vi "SaveDataFile.vi"(0 "Data Array":dbl[][](array[numeric])=[[1.0, 1.5e-10, 0.0, 0.0, 0.0], [2.0, 1.5e-10, 0.0, 0.0, 0.0], [3.0, 1.5e-10, 0.0, 0.0, 0.0], [4.0, 1.5e-10, 0.0, 0.0, 0.0]], 1 "Temperature":dbl=18.162352941176472, 3 "Humidity":dbl=25.207500000000007, 5 "no. of arrays":i32=5, 9 "Actual array lengths":i32=4, 11 "Error In":errorcluster, 12 "Array Titles":string="ProbeplanIndex Current PinholeFlag Capacitance Resistance", 13 "Strip Segment":string="Segment\t3T", 14 "Arrays format":string="%^g") -> (4 "Filename OUT":string="c-b1_Striptest_Segment_3T_1.dat", 6 "Pathname OUT":string="c:\\Users\\itk\\Documents\\itk-strip-sensor-data\\R0\\d\\c\\c-b1\\Striptest\\", 10 "Path + Filename OUT":string="c:\\Users\\itk\\Documents\\itk-strip-sensor-data\\R0\\d\\c\\c-b1\\Striptest\\c-b1_Striptest_Segment_3T_1.dat", 15 "Error Out":errorcluster)   [LabVIEW 2018]
uses:
  globals/QC_RunInformation.vi
  <vilib>/regexp/Match Regular Expression.xnode
panel:
  out "Data Array 3":dbl[](array[numeric])
  out "Data Array 2":dbl[](array[numeric])
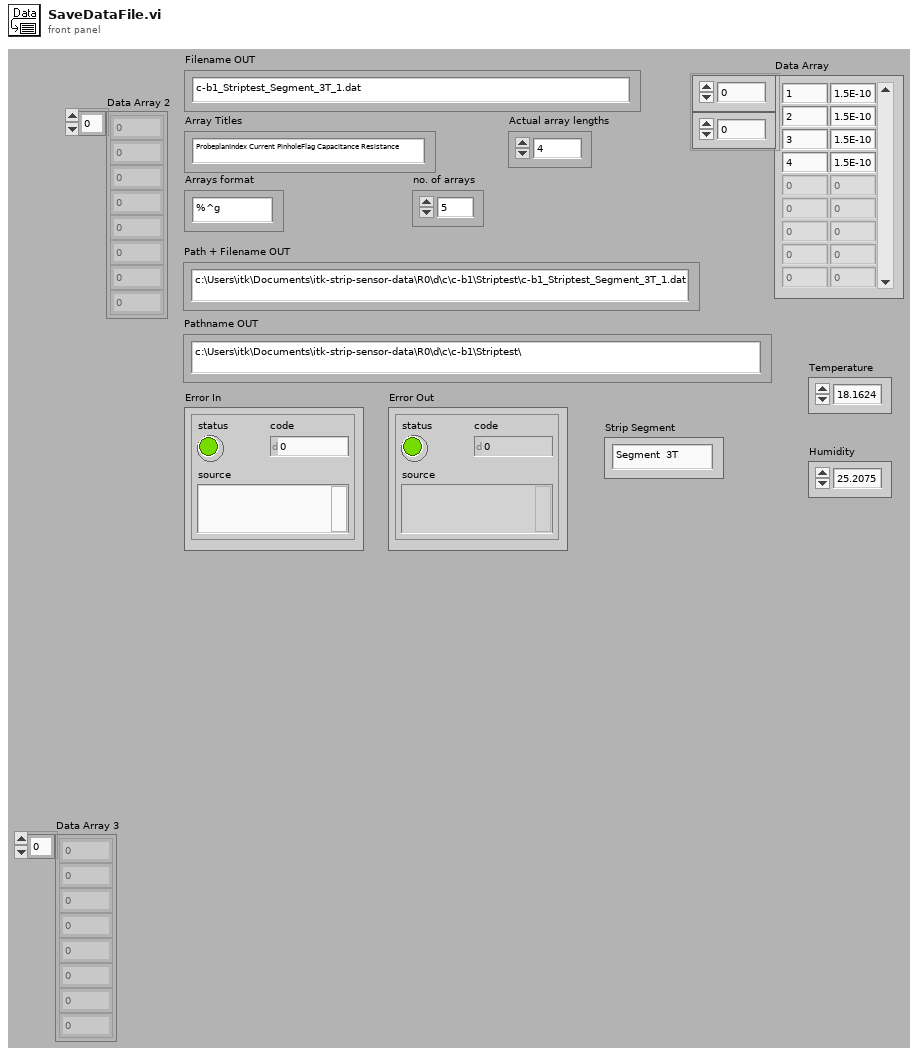
[diagram p1: front panel]
types:
  T1 = enum16{"open", "open or create", "create or replace", "create"}
  T2 = cluster{"Sensor Serial No.:":string, "Wafer Serial No.:":string, "Batch:":string, "Manufacturer:":string, "Device Category:":string, "Database Serial No.:":string, "Initiated:":string, "Test":string, "Instruments used:":string, "Probeplan used:":string, "End of Run comment:":string, "User:":string}
  T3 = cluster{"Institute":string, "Manufacturers":string[], "Devices":string[], "Serialnumbers Lookup DB":string, "Data directory":string, "Backup & screenshot directory":string, "List of known users":string[]}
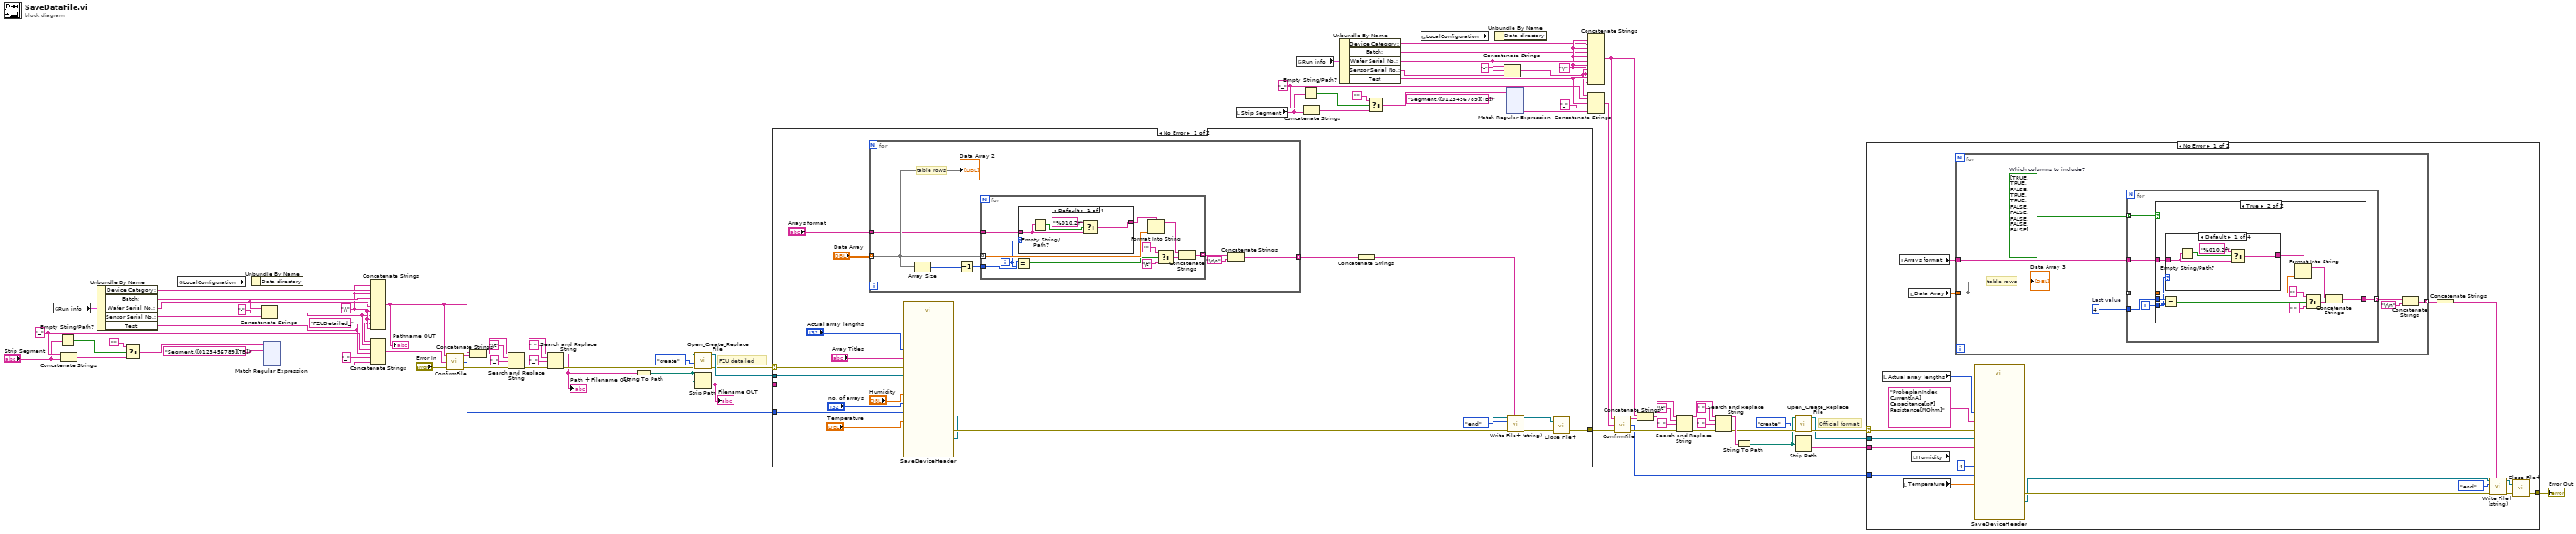
[diagram p0: block diagram]
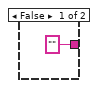
[diagram p2: hidden frame]
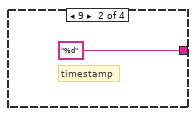
[diagram p3: hidden frame]
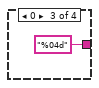
[diagram p4: hidden frame]
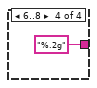
[diagram p5: hidden frame]
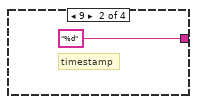
[diagram p7: hidden frame]
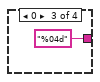
[diagram p8: hidden frame]
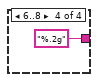
[diagram p9: hidden frame]
diagram:
  w29 = "_"
  w19 = "\\"
  w63 = "_"
  w72 = "\\"
  # "FZU detailed"
  # "Official format"
  n1 = global read "QC_RunInformation.vi" "Run info"() -> (w81:T2)
  n2 = Empty String/Path?(string/path="Strip Segment") -> (empty?=w65:bool)
  n3 = Concatenate Strings(w63, "Strip Segment") -> (w61:string)
  n4 = Unbundle By Name(w81) -> ("Device Category:"=w79:string, "Batch:"=w78:string, "Wafer Serial No.:"=w70:string, "Sensor Serial No.:"=w69:string, "Test"=w4:string)
  n5 = Select(t="", s=w65, f=w61) -> (s? t:f=w48:string)
  n6 = global read "QC_RunInformation.vi" "LocalConfiguration"() -> (w82:T3)
  n7 = Unbundle By Name(w82) -> ("Data directory"=w80:string)
  n8 = Concatenate Strings(w70, "-", w69) -> (w68:string)
  n9 = xnode "Match Regular Expression"("input string"=w48, "regular expression"="Segment.([0123456789][TB])") -> ("submatch 1"=w47:string)  [unwired: 4 in, 5 out]
  n10 = Concatenate Strings(w80, w72, w79, w72, w78, w72, w70, w72, w68, w72, w4, w72) -> (w66:string)
  "Pathname OUT" <- w66
  n11 = Concatenate Strings("FZUDetailed_" ("string"), w68, w63, w4, "_" ("string"), w47) -> (w67:string)
  n12 = call "ConfirmFile.vi"("Error In"="Error In", "Filename IN"=w67, "Pathname IN"=w66) -> ("Error Out"=w56:errorcluster, "RunNr"=w45:i32, "Filename:"=w60:string)
  n13 = Concatenate Strings(w66, w60) -> (w59:string)
  n14 = Search and Replace String(input string=w59, search string="\t" ("string"), replace string="_" ("substring (\"\")"), error in=w56) -> (result string=w53:string, error out=w55:errorcluster)  [unwired: 4 in, 2 out]
  n15 = Search and Replace String(input string=w53, search string=" " ("substring (\"\")"), replace string="_" ("substring (\"\")"), error in=w55) -> (result string=w52:string, error out=w54:errorcluster)  [unwired: 4 in, 2 out]
  "Path + Filename OUT" <- w52
  n16 = String To Path(string=w52) -> (path=w74:path)
  n17 = call <vilib>:"Open_Create_Replace File.vi"("error in (no error)"=w54, "function (open:0)"=T1."create", "file path"=w74) -> ("error out"=w73:errorcluster, "refnum"=w76:refnum<file>)  [unwired: 5 in, 2 out]
  n18 = Strip Path(path=w74) -> (name=w75:string)  [unwired: 1 out]
  "Filename OUT" <- w75
  n19 = case shown="No Error" w73 {
    selector: w73 -> [w101 w127]
    tunnel: w76 -> [w95 _]
    tunnel: w75 -> [w94 _]
    tunnel: [w90 w127] -> w5
    tunnel: w45 -> [w83 _]
    frame No Error {
      n20 = for {
        tunnel: "Data Array" -> [w108] mode=indexing
        tunnel: "Arrays format" -> [w103]
        tunnel: [w102] -> w85 mode=indexing
        # "table rows"
        n21 = Array Size(array=w108) -> (size(s)=w107:i32)
        n22 = Decrement(x=w107) -> (x-1=w106:i32)
        n23 = for {
          tunnel: w108 -> [w119] mode=indexing
          tunnel: w106 -> [w117]
          tunnel: [w111] -> w105 mode=indexing
          tunnel: w103 -> [w109]
          i -> [w110]
          n24 = Equal?(x=w117, y=w110) -> (x = y?=w116:bool)
          n25 = case shown="Default" w110 {
            tunnel: [w120 "%d" ("format string") "%04d" ("format string") "%.2g" ("format string")] -> w118
            tunnel: w109 -> [w121 _ _ _]
            frame Default {
              n26 = Empty String/Path?(string/path=w121) -> (empty?=w123:bool)
              n27 = Select(t="%010.2f", s=w123, f=w121) -> (s? t:f=w120:string)
            }
            frame 9 {
              # "timestamp"
            }
            frame 0 {
            }
            frame 6..8 {
            }
          }
          n28 = Format Into String(format string=w118, w119) -> (resulting string=w113:string)  [unwired: 2 in, 1 out]
          n29 = Select(t="" ("format string"), s=w116, f="\t" ("format string")) -> (s? t:f=w112:string)
          n30 = Concatenate Strings(w113, w112) -> (w111:string)
        }
        n31 = Concatenate Strings(w105, "\r\n") -> (w102:string)
        "Data Array 2" <- w108
      }
      n32 = call "SaveDeviceHeader.vi"("File Refnum in"=w95, "no. of arrays"="no. of arrays", "Array Lengths"="Actual array lengths", "Filename"=w94, "RunNr"=w83, "Array Titles"="Array Titles", "error in (no error)"=w101, "Temperature"="Temperature", "Humidity"="Humidity") -> ("File Refnum out"=w96:refnum<file>, "error out"=w97:errorcluster)  [unwired: 4 in, 1 out]
      n33 = Concatenate Strings(w85) -> (w84:string)
      n34 = call <vilib>:"Write File+ (string).vi"("string"=w84, "error in (no error)"=w97, "pos mode (rel. to end:1)"=enum16{"start", "end", "current"}."end", "refnum"=w96) -> ("error out"=w100:errorcluster, "dup refnum"=w98:refnum<file>)  [unwired: 3 in, 1 out]
      n35 = call <vilib>:"Close File+.vi"("error in (no error)"=w100, "refnum"=w98) -> ("error out"=w90:errorcluster)  [unwired: 3 in, 2 out]
    }
    frame Error {
    }
  }
  n36 = local read "Strip Segment"() -> (w1:string)
  n37 = global read "QC_RunInformation.vi" "Run info"() -> (w13:T2)
  n38 = Empty String/Path?(string/path=w1) -> (empty?=w27:bool)
  n39 = Concatenate Strings(w29, w1) -> (w30:string)
  n40 = Unbundle By Name(w13) -> ("Device Category:"=w15:string, "Batch:"=w16:string, "Wafer Serial No.:"=w21:string, "Sensor Serial No.:"=w22:string, "Test"=w25:string)
  n41 = Select(t="", s=w27, f=w30) -> (s? t:f=w43:string)
  n42 = global read "QC_RunInformation.vi" "LocalConfiguration"() -> (w12:T3)
  n43 = Unbundle By Name(w12) -> ("Data directory"=w14:string)
  n44 = Concatenate Strings(w21, "-", w22) -> (w23:string)
  n45 = xnode "Match Regular Expression"("input string"=w43, "regular expression"="Segment.([0123456789][TB])") -> ("submatch 1"=w44:string)  [unwired: 4 in, 5 out]
  n46 = Concatenate Strings(w14, w19, w15, w19, w16, w19, w21, w19, w23, w19, w25, w19) -> (w26:string)
  n47 = Concatenate Strings(w23, w29, w25, "_" ("string"), w44) -> (w24:string)
  n48 = call "ConfirmFile.vi"("Error In"=w5, "Filename IN"=w24, "Pathname IN"=w26) -> ("Error Out"=w35:errorcluster, "RunNr"=w7:i32, "Filename:"=w31:string)
  n49 = Concatenate Strings(w26, w31) -> (w32:string)
  n50 = Search and Replace String(input string=w32, search string="\t" ("string"), replace string="_" ("substring (\"\")"), error in=w35) -> (result string=w38:string, error out=w36:errorcluster)  [unwired: 4 in, 2 out]
  n51 = Search and Replace String(input string=w38, search string=" " ("substring (\"\")"), replace string="_" ("substring (\"\")"), error in=w36) -> (result string=w39:string, error out=w37:errorcluster)  [unwired: 4 in, 2 out]
  n52 = String To Path(string=w39) -> (path=w18:path)
  n53 = call <vilib>:"Open_Create_Replace File.vi"("error in (no error)"=w37, "function (open:0)"=T1."create", "file path"=w18) -> ("error out"=w10:errorcluster, "refnum"=w9:refnum<file>)  [unwired: 5 in, 2 out]
  n54 = Strip Path(path=w18) -> (name=w8:string)  [unwired: 1 out]
  n55 = case shown="No Error" w10 {
    selector: w10 -> [w146 w179]
    tunnel: w9 -> [w140 _]
    tunnel: w8 -> [w139 _]
    tunnel: [w138 w179] -> w6
    tunnel: w7 -> [w131 _]
    frame No Error {
      n56 = local read "Actual array lengths"() -> (w130:i32)
      n57 = local read "Arrays format"() -> (w134:string)
      n58 = local read "Temperature"() -> (w128:dbl)
      n59 = local read "Data Array"() -> (w135:dbl[][])
      n60 = local read "Humidity"() -> (w129:dbl)
      n61 = for {
        tunnel: w135 -> [w153] mode=indexing
        tunnel: w134 -> [w150]
        tunnel: [w149] -> w137 mode=indexing
        w147 = 4  # Last value
        w148 = bool[] [TRUE, TRUE, FALSE, TRUE, TRUE, FALSE, FALSE, FALSE, FALSE, FALSE]  # Which columns to include?
        # "table rows"
        n62 = for {
          tunnel: w153 -> [w159] mode=indexing
          tunnel: w147 -> [w158]
          tunnel: [w157] -> w152 mode=indexing
          tunnel: w150 -> [w155]
          tunnel: w148 -> [w154] mode=indexing
          i -> [w156]
          n63 = case shown="True" w154 {
            tunnel: w159 -> [_ w171]
            tunnel: w158 -> [_ w169]
            tunnel: ["" w163] -> w157
            tunnel: w156 -> [_ w162]
            tunnel: w155 -> [_ w161]
            frame False {
            }
            frame True {
              n64 = Equal?(x=w169, y=w162) -> (x = y?=w168:bool)
              n65 = case shown="Default" w162 {
                tunnel: [w172 "%d" ("format string") "%04d" ("format string") "%.2g" ("format string")] -> w170
                tunnel: w161 -> [w173 _ _ _]
                frame Default {
                  n66 = Empty String/Path?(string/path=w173) -> (empty?=w175:bool)
                  n67 = Select(t="%010.2f", s=w175, f=w173) -> (s? t:f=w172:string)
                }
                frame 9 {
                  # "timestamp"
                }
                frame 0 {
                }
                frame 6..8 {
                }
              }
              n68 = Format Into String(format string=w170, w171) -> (resulting string=w165:string)  [unwired: 2 in, 1 out]
              n69 = Select(t="" ("format string"), s=w168, f=" " ("format string")) -> (s? t:f=w164:string)
              n70 = Concatenate Strings(w165, w164) -> (w163:string)
            }
          }
        }
        n71 = Concatenate Strings(w152, "\r\n") -> (w149:string)
        "Data Array 3" <- w153
      }
      n72 = call "SaveDeviceHeader.vi"("File Refnum in"=w140, "no. of arrays"=4, "Array Lengths"=w130, "Filename"=w139, "RunNr"=w131, "Array Titles"="ProbeplanIndex Current[nA] Capacitance[pF] Resistance[MOhm]", "error in (no error)"=w146, "Temperature"=w128, "Humidity"=w129) -> ("File Refnum out"=w141:refnum<file>, "error out"=w142:errorcluster)  [unwired: 4 in, 1 out]
      n73 = Concatenate Strings(w137) -> (w136:string)
      n74 = call <vilib>:"Write File+ (string).vi"("string"=w136, "error in (no error)"=w142, "pos mode (rel. to end:1)"=enum16{"start", "end", "current"}."end", "refnum"=w141) -> ("error out"=w145:errorcluster, "dup refnum"=w143:refnum<file>)  [unwired: 3 in, 1 out]
      n75 = call <vilib>:"Close File+.vi"("error in (no error)"=w145, "refnum"=w143) -> ("error out"=w138:errorcluster)  [unwired: 3 in, 2 out]
    }
    frame Error {
    }
  }
  "Error Out" <- w6
